vi "OnOff Text.vi"(11 "Boolean":bool) -> (3 "On / Off":string)   [LabVIEW 2016]
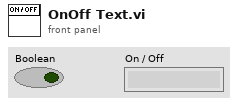
[diagram p1: front panel]
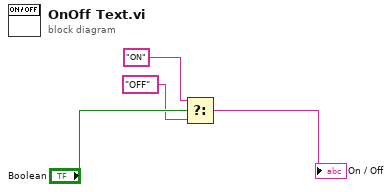
[diagram p0: block diagram]
diagram:
  n1 = Select(t="ON", s="Boolean", f="OFF") -> (s? t:f=→"On / Off":string)
